vi "multiFreqMultiSwitchMode.vi"(3 "步进频率":dbl=0.1, 4 "单片机串口":refnum<visa-resource-name>, 5 "步进距离":dbl=5.0, 6 "步进电机串口":refnum<visa-resource-name>) -> (0 "当前开关":dbl, 1 "当前频率":dbl, 2 "当前位置":dbl)   [LabVIEW 2018]
uses:
  <vilib>/Instr/_visa.llb/VISA Configure Serial Port (Instr).vi
  PCI8552B_32.dll
panel:
  in  "路径":path
  out "频率变化次数":dbl
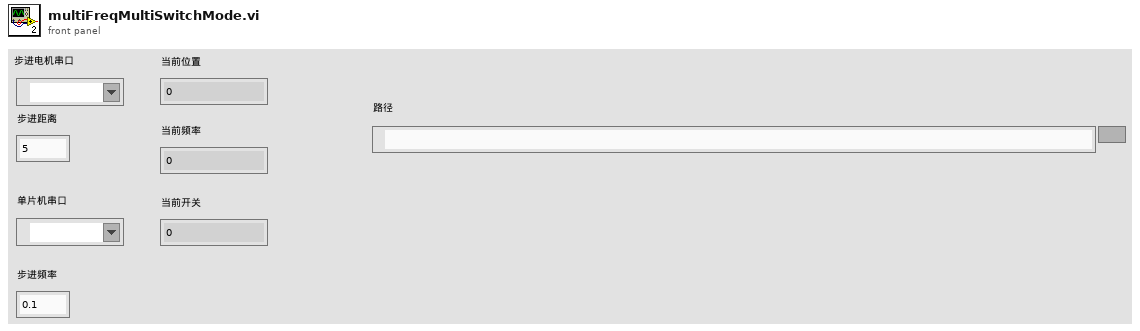
[diagram p1: front panel]
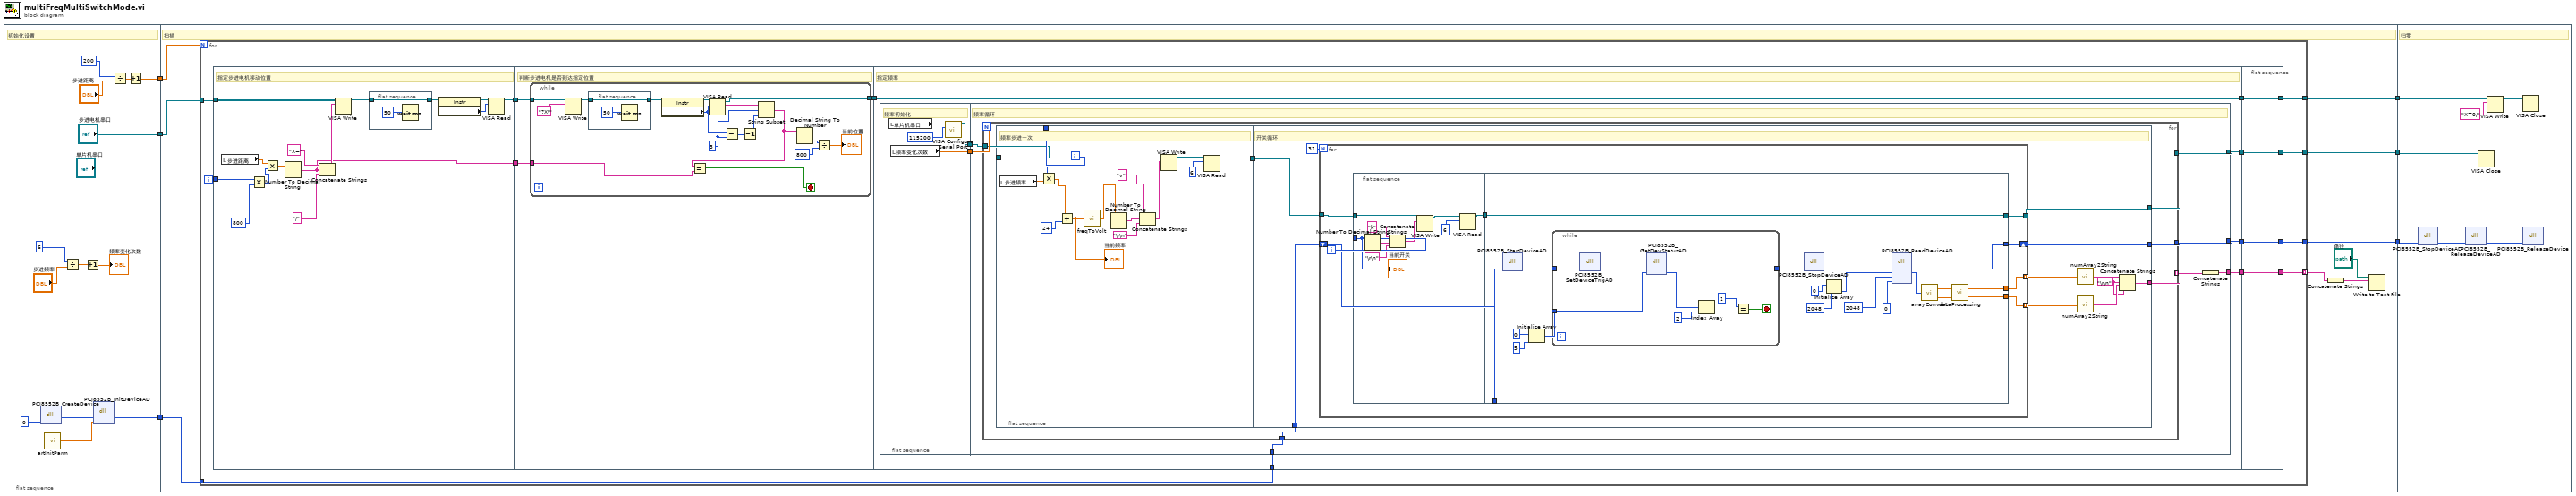
[diagram p0: block diagram]
diagram:
  n1 = flat-sequence {
    tunnel: [w16] -> w6
    tunnel: ["步进电机串口"] -> w5
    tunnel: [w7] -> w2
    tunnel: w6 -> [w28]
    tunnel: w5 -> [w27]
    tunnel: [w26] -> w4
    tunnel: [w25] -> w3
    tunnel: w2 -> [w24]
    tunnel: [w23] -> w1
    tunnel: w4 -> [w185]
    tunnel: w3 -> [w184]
    tunnel: w1 -> [w181]
    frame #0 {
      # "初始化设置"
      n2 = dll-call lib="PTH2abs E\nPersonal Fileç ç©¶çå­¦ä¹ 202002-202007ç ä¸ä¸å­¦æwork2020\nSARControllerSAR-ControllermainPCI8552B_32" fn="PCI8552B_CreateDevice" label="CreateDevice"("DeviceLgcID"=0) -> ("返回类型"=w9:i32)  [unwired: 4 in, 2 out]
      n3 = call "artInitParm.vi"() -> ("初始化参数"=w10:dbl[])
      n4 = Divide(x=6, y="步进频率") -> (x/y=w12:dbl)
      n5 = Increment(x=w12) -> (x+1=→"频率变化次数":dbl)
      n6 = dll-call lib="PTH2…abs E\nPersonal Fileç ”ç©¶ç”Ÿå­¦ä¹ 202002-202007ç ”ä¸€ä¸‹å­¦æœŸwork2020\nSARControllerSAR-ControllermainPCI8552B_32.DLL" fn="PCI8552B_InitDeviceAD" label="InitDeviceAD"("hDevice"=w9, "pADPara"=w10) -> ("hDevice"=w7:i32)  [unwired: 5 in, 2 out]
      n7 = Divide(x=200, y="步进距离") -> (x/y=w17:dbl)
      n8 = Increment(x=w17) -> (x+1=w16:dbl)
    }
    frame #1 {
      # "扫描"
      n9 = for {
        N: w28 -> [_]
        tunnel: w27 -> [w41]
        tunnel: [w36] -> w26
        tunnel: [w34] -> w25
        tunnel: w24 -> [w33]
        tunnel: [w31] -> w23
        tunnel: [w29] -> w22 mode=indexing
        i -> [w42]
        n10 = flat-sequence "平铺式顺序结构" {
          tunnel: w42 -> [w56]
          tunnel: w41 -> [w52]
          tunnel: [w45] -> w40
          tunnel: [w43] -> w39
          tunnel: w40 -> [w62]
          tunnel: w39 -> [w61]
          tunnel: [w60] -> w37
          tunnel: [w88] -> w38
          tunnel: w37 -> [w88]
          tunnel: [w85] -> w35
          tunnel: w33 -> [w84]
          tunnel: [w83] -> w32
          tunnel: [w82] -> w30
          tunnel: w38 -> [w180]
          tunnel: [w180] -> w36
          tunnel: w35 -> [w179]
          tunnel: [w179] -> w34
          tunnel: w32 -> [w178]
          tunnel: [w178] -> w31
          tunnel: w30 -> [w177]
          tunnel: [w177] -> w29
          frame #0 {
            # "指定步进电机移动位置"
            n11 = local read "步进距离"() -> (w55:dbl)
            n12 = Multiply(x=w56, y=800) -> (x*y=w54:i32)
            n13 = Multiply(x=w55, y=w54) -> (x*y=w53:dbl)
            n14 = Number To Decimal String(number=w53) -> (decimal integer string=w43:string)  [unwired: 1 in]
            n15 = Concatenate Strings("X=", w43, "/") -> (w44:string)
            n16 = VISA Write(VISA resource name=w52, write buffer=w44) -> (VISA resource name out=w49:refnum<visa-resource-name>)  [unwired: 1 in, 2 out]
            n17 = flat-sequence {
              tunnel: w49 -> [w58]
              tunnel: [w58] -> w48
              frame #0 {
                n18 = Wait (ms)(milliseconds to wait=50) -> ()  [unwired: 1 out]
              }
            }
            n19 = property class="Instr"(reference=w48) -> (reference out=w47:refnum<visa-resource-name>, "Serial Settings:Number of Bytes at Serial Port"=w46:u32)  [unwired: 1 in, 1 out]
            n20 = VISA Read(VISA resource name=w47, byte count=w46) -> (VISA resource name out=w45:refnum<visa-resource-name>)  [unwired: 1 in, 3 out]
          }
          frame #1 {
            # "判断步进电机是否到达指定位置"
            n21 = while {
              tunnel: w62 -> [w79]
              tunnel: w61 -> [w69]
              tunnel: [w67] -> w60
              stop <- w68 stop-if-true
              w72 = 3
              n22 = VISA Write(VISA resource name=w79, write buffer="?X/") -> (VISA resource name out=w77:refnum<visa-resource-name>)  [unwired: 1 in, 2 out]
              n23 = flat-sequence {
                tunnel: w77 -> [w80]
                tunnel: [w80] -> w76
                frame #0 {
                  n24 = Wait (ms)(milliseconds to wait=50) -> ()  [unwired: 1 out]
                }
              }
              n25 = property class="Instr"(reference=w76) -> (reference out=w75:refnum<visa-resource-name>, "Serial Settings:Number of Bytes at Serial Port"=w73:u32)  [unwired: 1 in, 1 out]
              n26 = VISA Read(VISA resource name=w75, byte count=w73) -> (VISA resource name out=w67:refnum<visa-resource-name>, read buffer=w74:string)  [unwired: 1 in, 2 out]
              n27 = Subtract(x=w73, y=w72) -> (x-y=w71:u32)
              n28 = Decrement(x=w71) -> (x-1=w70:u32)
              n29 = String Subset(string=w74, offset (0)=w72, length (rest)=w70) -> (substring=w66:string)
              n30 = Equal?(x=w66, y=w69) -> (x = y?=w68:bool)
              n31 = Decimal String To Number(string=w66) -> (number=w65:i32)  [unwired: 2 in, 1 out]
              n32 = Divide(x=w65, y=800) -> (x/y=→"当前位置":dbl)
            }
          }
          frame #2 {
            # "指定频率"
            n33 = flat-sequence {
              tunnel: [w90] -> w87
              tunnel: [w89] -> w86
              tunnel: w87 -> [w99]
              tunnel: w86 -> [w98]
              tunnel: [w97] -> w85
              tunnel: w84 -> [w96]
              tunnel: [w95] -> w83
              tunnel: [w93] -> w82
              frame #0 {
                # "频率初始化"
                n34 = local read "单片机串口"() -> (w91:refnum<visa-resource-name>)
                n35 = local read "频率变化次数"() -> (w90:dbl)
                n36 = call-poly "VISA Configure Serial Port"("VISA resource name"=w91, "baud rate (9600)"=115200) -> ("VISA resource name out"=w89:refnum<visa-resource-name>)  [unwired: 12 in, 1 out]
              }
              frame #1 {
                # "频率循环"
                n37 = for {
                  N: w99 -> [_]
                  tunnel: w98 -> [w105]
                  tunnel: [w103] -> w97
                  tunnel: w96 -> [w102]
                  tunnel: [w101] -> w95
                  tunnel: [w100] -> w94 mode=indexing
                  i -> [w106]
                  n38 = flat-sequence {
                    tunnel: w106 -> [w120]
                    tunnel: w105 -> [w116]
                    tunnel: [w112] -> w104
                    tunnel: w104 -> [w130]
                    tunnel: [w129] -> w103
                    tunnel: w102 -> [w128]
                    tunnel: [w127] -> w101
                    tunnel: [w122] -> w100
                    frame #0 {
                      # "频率步进一次"
                      n39 = local read "步进频率"() -> (w119:dbl)
                      n40 = Multiply(x=w120, y=w119) -> (x*y=w118:dbl)
                      n41 = Add(x=w118, y=24) -> (x+y=w107:dbl)
                      "当前频率" <- w107
                      n42 = call "freqToVolt.vi"("频率"=w107) -> ("电压"=w110:dbl)
                      n43 = Number To Decimal String(number=w110) -> (decimal integer string=w114:string)  [unwired: 1 in]
                      n44 = Concatenate Strings("v", w114, "\r\n") -> (w111:string)
                      n45 = VISA Write(VISA resource name=w116, write buffer=w111) -> (VISA resource name out=w109:refnum<visa-resource-name>)  [unwired: 1 in, 2 out]
                      n46 = VISA Read(VISA resource name=w109, byte count=6) -> (VISA resource name out=w112:refnum<visa-resource-name>)  [unwired: 1 in, 3 out]
                    }
                    frame #1 {
                      w121 = "\r\n"
                      # "开关循环"
                      n47 = for {
                        N: 31 -> [_]
                        tunnel: w130 -> [w139]
                        tunnel: [w138] -> w129
                        shift-right: [w135] -> w127
                        shift-left: w128 -> [w134]
                        tunnel: [w133] -> w126 mode=indexing
                        tunnel: [w132] -> w125 mode=indexing
                        i -> [w137]
                        n48 = flat-sequence {
                          tunnel: w139 -> [w148]
                          tunnel: w137 -> [w140]
                          tunnel: [w143] -> w136
                          tunnel: [w167] -> w138
                          tunnel: w136 -> [w167]
                          tunnel: [w149] -> w135
                          tunnel: w134 -> [w150]
                          tunnel: [w161] -> w133
                          tunnel: [w160] -> w132
                          frame #0 {
                            n49 = Number To Decimal String(number=w140) -> (decimal integer string=w147:string)  [unwired: 1 in]
                            n50 = Concatenate Strings("k", w147, "\r\n") -> (w144:string)
                            n51 = VISA Write(VISA resource name=w148, write buffer=w144) -> (VISA resource name out=w142:refnum<visa-resource-name>)  [unwired: 1 in, 2 out]
                            n52 = VISA Read(VISA resource name=w142, byte count=6) -> (VISA resource name out=w143:refnum<visa-resource-name>)  [unwired: 1 in, 3 out]
                            "当前开关" <- w140
                          }
                          frame #1 {
                            n53 = dll-call lib="PTH2…abs E\nPersonal Fileç ”ç©¶ç”Ÿå­¦ä¹ 202002-202007ç ”ä¸€ä¸‹å­¦æœŸwork2020\nSARControllerSAR-ControllermainPCI8552B_32.DLL" fn="PCI8552B_StartDeviceAD" label="StartDeviceAD"("hDevice"=w150) -> ("hDevice"=w151:i32)  [unwired: 4 in, 2 out]
                            n54 = Initialize Array(0, 5) -> (w156:i32[])
                            n55 = while {
                              tunnel: w151 -> [w171]
                              tunnel: w156 -> [w176]
                              tunnel: [w169] -> w153
                              stop <- w168 stop-if-true
                              n56 = dll-call lib="PTH2…abs E\nPersonal Fileç ”ç©¶ç”Ÿå­¦ä¹ 202002-202007ç ”ä¸€ä¸‹å­¦æœŸwork2020\nSARControllerSAR-ControllermainPCI8552B_32.DLL" fn="PCI8552B_SetDeviceTrigAD" label="SetDeviceTrigAD"("hDevice"=w171) -> ("hDevice"=w170:i32)  [unwired: 4 in, 2 out]
                              n57 = dll-call lib="PTH2…abs E\nPersonal Fileç ”ç©¶ç”Ÿå­¦ä¹ 202002-202007ç ”ä¸€ä¸‹å­¦æœŸwork2020\nSARControllerSAR-ControllermainPCI8552B_32.DLL" fn="PCI8552B_GetDevStatusAD" label="GetDevStatusAD"("hDevice"=w170, "ADStatus"=w176) -> ("hDevice"=w169:i32, "ADStatus"=w172:i32[])  [unwired: 4 in, 2 out]
                              n58 = Index Array(array=w172, index=2) -> (element=w174:i32)
                              n59 = Equal?(x=1, y=w174) -> (x = y?=w168:bool)
                            }
                            n60 = dll-call lib="PTH2…abs E\nPersonal Fileç ”ç©¶ç”Ÿå­¦ä¹ 202002-202007ç ”ä¸€ä¸‹å­¦æœŸwork2020\nSARControllerSAR-ControllermainPCI8552B_32.DLL" fn="PCI8552B_StopDeviceAD" label="StopDeviceAD"("hDevice"=w153) -> ("hDevice"=w152:i32)  [unwired: 4 in, 2 out]
                            n61 = Initialize Array(u16 0 ("y"), 2048 ("y")) -> (w166:u16[])
                            n62 = dll-call lib="PTH2…abs E\nPersonal Fileç ”ç©¶ç”Ÿå­¦ä¹ 202002-202007ç ”ä¸€ä¸‹å­¦æœŸwork2020\nSARControllerSAR-ControllermainPCI8552B_32.DLL" fn="PCI8552B_ReadDeviceAD" label="ReadDeviceAD"("hDevice"=w152, "pADBuffer"=w166, "nReadSizeWords"=2048 ("y"), "nRetSizeWords"=u16 0 ("y")) -> ("hDevice"=w149:i32, "pADBuffer"=w157:u16[])  [unwired: 6 in, 2 out]
                            n63 = call "arrayConvert.vi"("输入数组"=w157) -> ("ch0"=w159:dbl[], "ch1"=w158:dbl[])
                            n64 = call "dataProcessing.vi"("参考信号"=w158, "中频信号"=w159) -> ("mean_Q"=w160:dbl, "mean_I"=w161:dbl)
                          }
                        }
                      }
                      n65 = call "numArray2String.vi"("输入数组"=w125) -> ("输出字符串"=w123:string)
                      n66 = call "numArray2String.vi"("输入数组"=w126) -> ("输出字符串"=w124:string)
                      n67 = Concatenate Strings(w124, w121, w123, w121) -> (w122:string)
                    }
                  }
                }
                n68 = Concatenate Strings(w94) -> (w93:string)
              }
            }
          }
          frame #3 {
          }
        }
      }
      n69 = Concatenate Strings(w22) -> (w21:string)
      n70 = Write to Text File(file (use dialog)="路径", text=w21) -> ()  [unwired: 2 in, 3 out]
    }
    frame #2 {
      # "归零"
      n71 = dll-call lib="PTH2…abs E\nPersonal Fileç ”ç©¶ç”Ÿå­¦ä¹ 202002-202007ç ”ä¸€ä¸‹å­¦æœŸwork2020\nSARControllerSAR-ControllermainPCI8552B_32.DLL" fn="PCI8552B_StopDeviceAD" label="StopDeviceAD"("hDevice"=w181) -> ("hDevice"=w182:i32)  [unwired: 4 in, 2 out]
      n72 = dll-call lib="PTH2…abs E\nPersonal Fileç ”ç©¶ç”Ÿå­¦ä¹ 202002-202007ç ”ä¸€ä¸‹å­¦æœŸwork2020\nSARControllerSAR-ControllermainPCI8552B_32.DLL" fn="PCI8552B_ReleaseDeviceAD" label="ReleaseDeviceAD"("hDevice"=w182) -> ("hDevice"=w183:i32)  [unwired: 4 in, 2 out]
      n73 = VISA Close(VISA resource name=w184) -> ()  [unwired: 1 in, 1 out]
      n74 = VISA Write(VISA resource name=w185, write buffer="X=0/") -> (VISA resource name out=w187:refnum<visa-resource-name>)  [unwired: 1 in, 2 out]
      n75 = VISA Close(VISA resource name=w187) -> ()  [unwired: 1 in, 1 out]
      n76 = dll-call lib="PTH2…abs E\nPersonal Fileç ”ç©¶ç”Ÿå­¦ä¹ 202002-202007ç ”ä¸€ä¸‹å­¦æœŸwork2020\nSARControllerSAR-ControllermainPCI8552B_32.DLL" fn="PCI8552B_ReleaseDevice" label="ReleaseDevice"("hDevice"=w183) -> ()  [unwired: 5 in, 2 out]
    }
  }
